vi "Obtain Session.vi"(0 "PropertyObject":refnum<k7>, 5 "PropertyObjectFile":refnum<k7>, 11 "error in (no error)":errorcluster) -> (4 "Session Handle":T1, 15 "error out":errorcluster)   [LabVIEW 2020, in "HTS.lvlib" / "VariableContainer.lvclass"]
doc: "This function initializes the measurement\n\nPass the function a name to obtain an active measurement handle"
uses:
  VariableContainer.lvclass
  Typedefs/Session Handle.ctl
  C:/Program Files (x86)/National Instruments/LabVIEW 2020/user.lib/_Session Fwk/Session - Root.lvclass
  VariableContainer.lvclass/VariableContainer.ctl
  <userlib>/_Session Fwk/Session - Root.lvclass
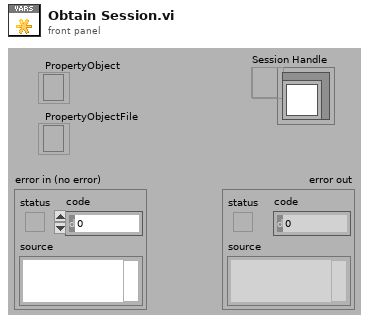
[diagram p1: front panel]
types:
  T1 = typedef "HTS.lvlib/VariableContainer.lvclass/Session Handle.ctl" = refnum<data-value>
  T2 = typedef "Session - Root.lvclass/Session Handle.ctl" = refnum<data-value>
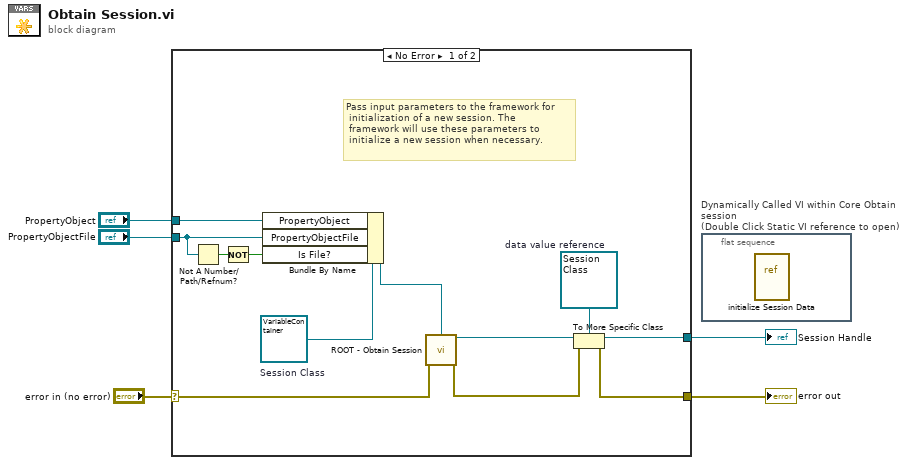
[diagram p0: block diagram]
diagram:
  n1 = case shown="No Error" "error in (no error)" {
    selector: "error in (no error)" -> [w17 w18]
    tunnel: [w14 w18] -> w4
    tunnel: [w16 _] -> w3
    tunnel: "PropertyObject" -> [w11 _]
    tunnel: "PropertyObjectFile" -> [w8 _]
    frame No Error {
      w9 = refnum<data-value> refnum  # data value reference
      w10 = refnum<class "VariableContainer.lvclass"> refnum  # Session Class
      # "Pass input parameters to the framework for\n initialization of a new session. The\n framework will use these parameters to\n initialize a new session when necessary."
      n2 = Not A Number/Path/Refnum?(number/path/refnum=w8) -> (NaN/Path/Refnum?=w7:bool)
      n3 = Not(x=w7) -> (.not. x?=w6:bool)
      n4 = Bundle By Name(cluster=w10, "PropertyObject"=w11, "PropertyObjectFile"=w8, "Is File?"=w6) -> (w12:refnum<class "VariableContainer.lvclass">)
      n5 = call <userlib>:"ROOT - Obtain Session.vi"("OBJ - Session"=w12, "error in (no error)"=w17) -> ("Session Handle"=w13:T2, "error out"=w15:errorcluster)  [unwired: 11 in, 1 out]
      n6 = To More Specific Class(target class=w9, reference=w13, error in=w15) -> (specific class reference=w16:refnum<data-value>, error out=w14:errorcluster)
    }
    frame Error {
    }
  }
  "error out" <- w4
  "Session Handle" <- w3
  n7 = flat-sequence "Dynamically Called VI within Core Obtain session\n(Double Click Static VI reference to open)" {
    frame #0 {
      n8 = vi-ref "initialize Session Data.vi"() -> ()  [unwired: 1 out]
    }
  }
